vi "5.10 WebCam Demovi.vi"() -> ()   [LabVIEW 2010]
uses:
  4-High Neurons/4.0-Timing Badass.ctl
  <vilib>/userDefined/High Color/IMAQdx.ctl
  5.10 Algorithm Parameters and Controls.ctl
  <vilib>/Analysis/Matrix/Numeric/Conversions/Array To Matrix - RA2.vi
  <vilib>/Analysis/Matrix/Numeric/Conversions/Array To Matrix - RA.vi
  <vilib>/vision/driver/NI_Vision_Acquisition_Software.lvlib
  <vilib>/Analysis/Matrix/NI_Matrix.lvlib
panel:
  in  "Rotation of Camera":dbl[][](array[numeric])=[[1.0, 0.0, 0.0], [0.0, 1.0, 0.0], [0.0, 0.0, 1.0]]
  in  "Location of Camera":dbl[](array[numeric])=[0.0, 0.0, 0.0]
  out "XY Graph":cluster{dbl[], dbl[]}[](graph)
  out "Randy Blue Actual":dbl
  out "Larry Blue Actual":dbl
  in  "Larry Exposure":dbl=0.02
  out "Larry Blue Threshold Used":dbl
  in  "Randy Exposure":dbl=0.02
  out "Randy B/W Overlay (R4)":T1(plugin-control)
  out "Randy Color Overlay (R5)":T1(plugin-control)
  in  "Randy Blue Threshold":i32=120
  out "Larry Color Overlay (L5)":T1(plugin-control)
  out "Larry B/W Overlay (L4)":T1(plugin-control)
  out "Larry Re-Map (L3)":T1(plugin-control)
  out "Randy Plane (R2)":T1(plugin-control)
  out "Larry Plane (L2)":T1(plugin-control)
  out "Randy Resample (R1)":T1(plugin-control)
  out "Larry Resample (L1)":T1(plugin-control)
  out "Raw Randy (L0)":T1(plugin-control)
  in  "Larry Blue Threshold":i32=120
  in  "Gains and Parameters":T2={"Control Gain"=0.5, "Line Setpoint in Pixels"=2.0, "Low Pass Gain"=1.2, "Image Low Pass Gain"=0.2, "Line Fullness Setpoint"=0.1, "Line Fullness Std"=0.2, "Max Filter Mod"=-10.0}
  out "Raw Larry (L0)":T1(plugin-control)
  in  "Larry":T3
  in  "Randy":T3
  out "Randy Re-Map (R3)":T1(plugin-control)
  out "Super Heart Beat":T4
  in  "Resample Scaling":i32=20 min=1 max=400 step=1
  in  "stop":bool
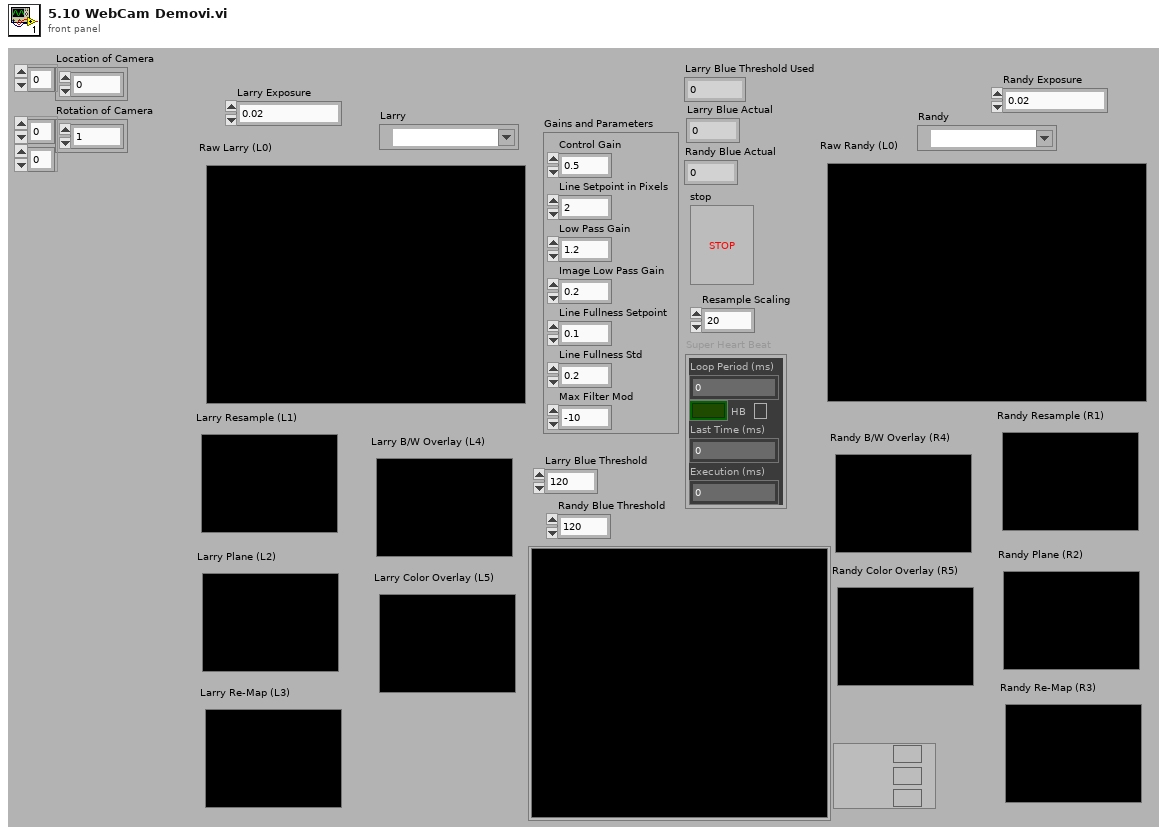
[diagram p1: front panel]
types:
  T1 = typedef "IMAQ Image.ctl" = refnum<image>
  T2 = typedef "5.10 Algorithm Parameters and Controls.ctl" = cluster{"Control Gain":dbl, "Line Setpoint in Pixels":dbl, "Low Pass Gain":dbl, "Image Low Pass Gain":dbl, "Line Fullness Setpoint":dbl, "Line Fullness Std":dbl, "Max Filter Mod":dbl}
  T3 = typedef "IMAQdx.ctl" = refnum<k21>
  T4 = typedef "4.0-Timing Badass.ctl" = cluster{"Loop Period (ms)":u32, "HB":bool, "Last Time (ms)":u32, "Execution (ms)":u32}
  T5 = typedef "5.10 Buffers Cluster.ctl" = cluster{"IMAQ Session":T3, "Buffer 0: Raw":T1, "Buffer 1: Resample":T1, "Buffer 2: Plane Extraction":T1, "Buffer 3: Re-mapping":T1, "Buffer 4: Overlay B/W":T1, "Buffer 5: Overlay Color":T1, "Buffer 6: Mask":T1, "Buffer 7: Masked Resample":T1}
  T6 = typedef "NI_Matrix.lvlib/RealMatrix.ctl" = dbl[][]
  T7 = typedef "6.10.1 LineDef.ctl" = cluster{"Vector 1 X":dbl, "Vector 1 Y":dbl, "Vector 2 X":dbl, "Vector 2 Y":dbl, "Center X":dbl, "Center Y":dbl}
  T8 = cluster{"Drive Angles":dbl[], "Drive Speeds":dbl[]}
  T9 = cluster{"Drive Angles":dbl[], "Drive Speeds":dbl[]}[]
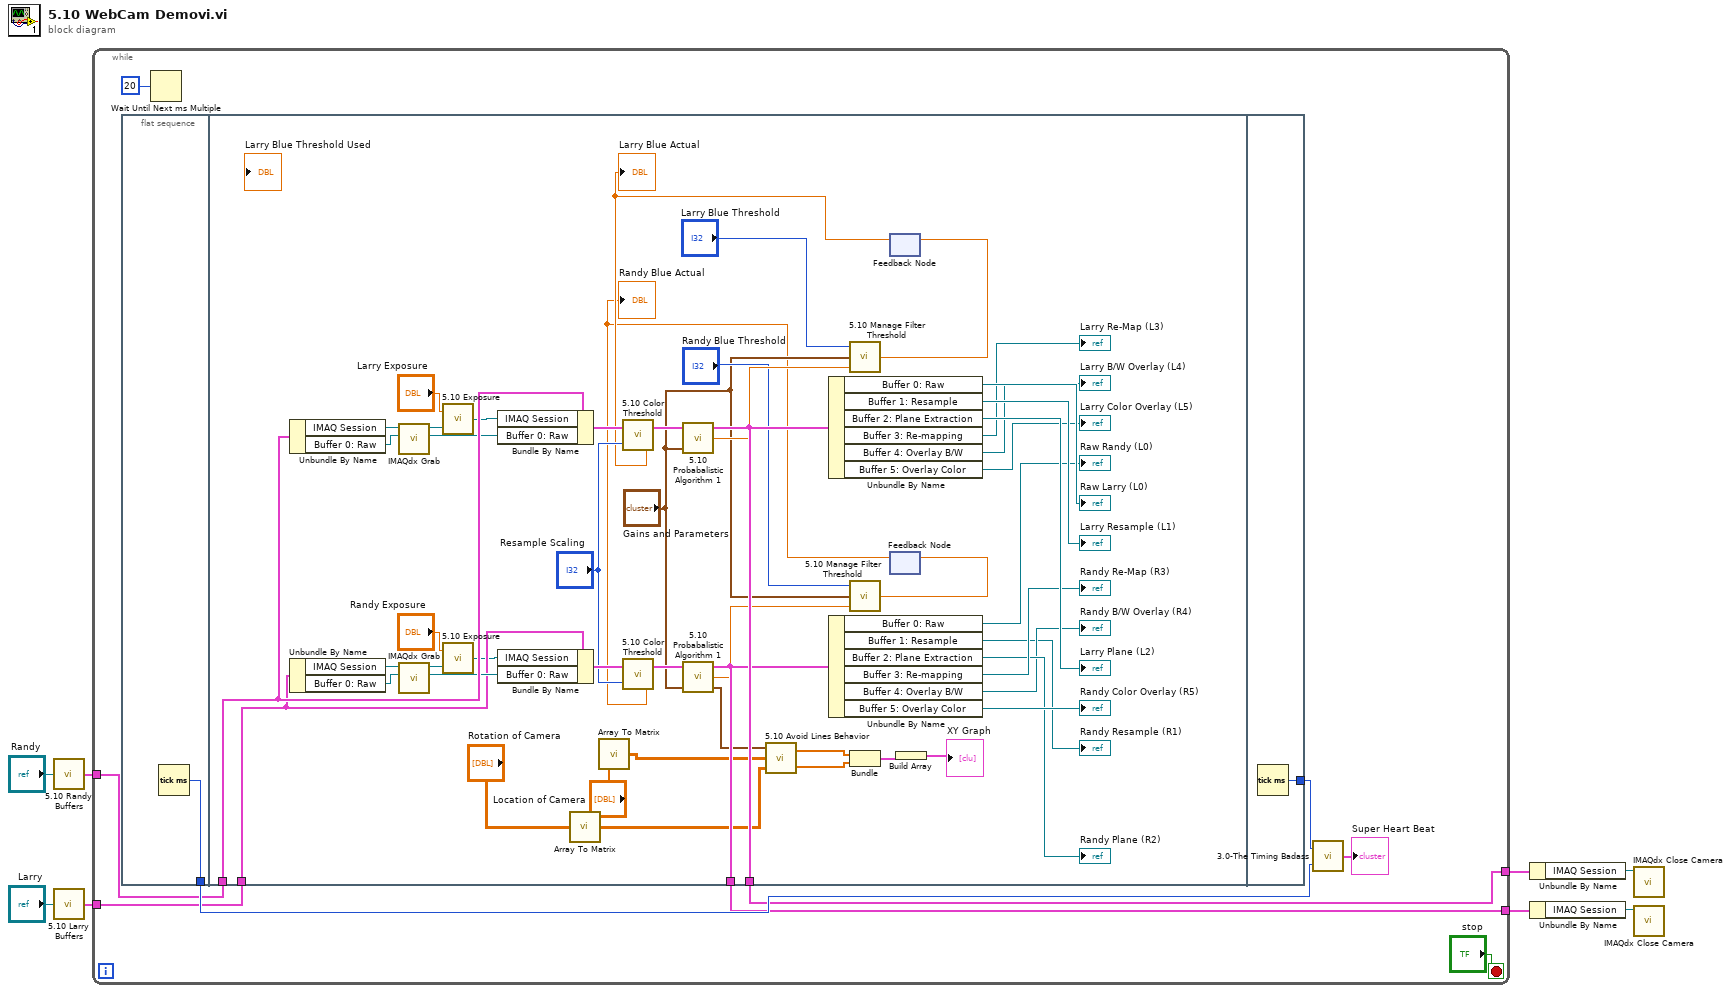
[diagram p0: block diagram]
diagram:
  n1 = call "5.10 Randy Buffers.vi"("Randy"="Randy") -> ("Randy Buffers"=w6:T5)
  n2 = call "5.10 Larry Buffers.vi"("Larry"="Larry") -> ("Larry Buffers"=w2:T5)
  n3 = while {
    tunnel: w6 -> [w12]
    tunnel: [w11] -> w5
    tunnel: w2 -> [w10]
    tunnel: [w9] -> w1
    stop <- "stop" stop-if-true
    n4 = flat-sequence {
      tunnel: [w18] -> w15
      tunnel: w12 -> [w67]
      tunnel: [w62] -> w11
      tunnel: w10 -> [w58]
      tunnel: [w55] -> w9
      tunnel: [w70] -> w16
      frame #0 {
        n5 = Tick Count (ms)() -> (millisecond timer value=w18:u32)
      }
      frame #1 {
        n6 = Unbundle By Name(w67) -> ("IMAQ Session"=w66:T3, "Buffer 0: Raw"=w65:T1)
        n7 = Unbundle By Name(w58) -> ("IMAQ Session"=w59:T3, "Buffer 0: Raw"=w60:T1)
        n8 = call <vilib>:"IMAQdx Grab.vi"("Image In"=w65, "Session In"=w66) -> ("Image Out"=w64:T1, "Session Out"=w38:T3)  [unwired: 6 in, 2 out]
        n9 = call <vilib>:"IMAQdx Grab.vi"("Image In"=w60, "Session In"=w59) -> ("Image Out"=w61:T1, "Session Out"=w39:T3)  [unwired: 6 in, 2 out]
        n10 = call "5.10 Exposure.vi"("Session In"=w38, "Exposure"="Larry Exposure") -> ("Session Out"=w37:T3)
        n11 = call "5.10 Exposure.vi"("Session In"=w39, "Exposure"="Randy Exposure") -> ("Session Out"=w41:T3)
        n12 = Bundle By Name(cluster=w67, "IMAQ Session"=w37, "Buffer 0: Raw"=w64) -> (w63:T5)
        n13 = Bundle By Name(cluster=w58, "IMAQ Session"=w41, "Buffer 0: Raw"=w61) -> (w56:T5)
        n14 = call-poly <vilib>:"Array To Matrix.vi"("Real 2D Array"="Rotation of Camera") -> ("Real Matrix"=w23:T6)
        n15 = call-poly <vilib>:"Array To Matrix.vi"("Real 1D Array"="Location of Camera") -> ("Real Matrix (Column Vector)"=w24:T6)
        n16 = feedback #1() -> (w33:dbl)  [unwired: 1 in]
        "Larry Blue Actual" <- w33
        n17 = call "5.10 Color Threshold.vi"("Input Fuzzy Blue Threshold"=w33, "Resample Scaling"="Resample Scaling", "Buffers In"=w63) -> ("Buffers Out"=w69:T5)
        n18 = call "5.10 Probabalistic Algorithm 1.vi"("Gains and Parameters"="Gains and Parameters", "Buffers Cluster In"=w69) -> ("Output Control Signal"=w35:dbl, "Buffers Cluster Out"=w62:T5)  [unwired: 1 in, 1 out]
        n19 = Unbundle By Name(w62) -> ("Buffer 0: Raw"=→"Raw Larry (L0)":T1, "Buffer 1: Resample"=→"Larry Resample (L1)":T1, "Buffer 2: Plane Extraction"=→"Larry Plane (L2)":T1, "Buffer 3: Re-mapping"=→"Larry Re-Map (L3)":T1, "Buffer 4: Overlay B/W"=→"Larry B/W Overlay (L4)":T1, "Buffer 5: Overlay Color"=→"Larry Color Overlay (L5)":T1)
        n20 = call "5.10 Manage Filter Threshold.vi"("Output Control Signal"=w35, "Gains and Parameters"="Gains and Parameters", "Filter Control"="Larry Blue Threshold") -> ("Filter Value Output"=w34:dbl)
        n21 = feedback-in #1(w34) -> ()
        n22 = feedback #2() -> (w28:dbl)  [unwired: 1 in]
        "Randy Blue Actual" <- w28
        n23 = call "5.10 Color Threshold.vi"("Input Fuzzy Blue Threshold"=w28, "Resample Scaling"="Resample Scaling", "Buffers In"=w56) -> ("Buffers Out"=w57:T5)
        n24 = call "5.10 Probabalistic Algorithm 1.vi"("Gains and Parameters"="Gains and Parameters", "Buffers Cluster In"=w57) -> ("Line Def"=w27:T7, "Output Control Signal"=w30:dbl, "Buffers Cluster Out"=w55:T5)  [unwired: 1 in]
        n25 = call "5.10 Avoid Lines Behavior.vi"("Rotation of Camera"=w23, "Location of Camera"=w24, "Line Def"=w27) -> ("Drive Speeds"=w21:dbl[], "Drive Angles"=w22:dbl[])
        n26 = Unbundle By Name(w55) -> ("Buffer 0: Raw"=→"Raw Randy (L0)":T1, "Buffer 1: Resample"=→"Randy Resample (R1)":T1, "Buffer 2: Plane Extraction"=→"Randy Plane (R2)":T1, "Buffer 3: Re-mapping"=→"Randy Re-Map (R3)":T1, "Buffer 4: Overlay B/W"=→"Randy B/W Overlay (R4)":T1, "Buffer 5: Overlay Color"=→"Randy Color Overlay (R5)":T1)
        n27 = call "5.10 Manage Filter Threshold.vi"("Output Control Signal"=w30, "Gains and Parameters"="Gains and Parameters", "Filter Control"="Randy Blue Threshold") -> ("Filter Value Output"=w29:dbl)
        n28 = Bundle("Drive Angles"=w22, "Drive Speeds"=w21) -> (w20:T8)  [unwired: 1 in]
        n29 = feedback-in #2(w29) -> ()
        n30 = Build Array(w20) -> (→"XY Graph":T9)
      }
      frame #2 {
        n31 = Tick Count (ms)() -> (millisecond timer value=w70:u32)
      }
    }
    n32 = Wait Until Next ms Multiple(millisecond multiple=u32 20) -> ()  [unwired: 1 out]
    n33 = call "3.0-The Timing Badass.vi"("Start"=w15, "End"=w16) -> ("Super Heart Beat"=→"Super Heart Beat":T4)
  }
  n34 = Unbundle By Name(w5) -> ("IMAQ Session"=w4:T3)
  n35 = Unbundle By Name(w1) -> ("IMAQ Session"=w3:T3)
  n36 = call <vilib>:"IMAQdx Close Camera.vi"("Session In"=w4) -> ()  [unwired: 10 in, 1 out]
  n37 = call <vilib>:"IMAQdx Close Camera.vi"("Session In"=w3) -> ()  [unwired: 10 in, 1 out]
